vi "Unit Test FGV slit.vi"() -> ()   [LabVIEW 2013]
doc: "Use this template to build a producer/consumer design pattern with events to produce queue items. Use this design pattern instead of the User Interface Event Handler pattern for user interfaces when you want to execute code asynchronously in response to an event without slowing the user interface responsiveness."
uses:
  FGV Slit Data.ctl
  <userlib>/GCSLabView/Low Level/General command.llb/Controller names.ctl
  Action Slit.ctl
  <userlib>/GCSLabView/Low Level/General command.llb/Global2 (Array).vi
panel:
  out "System":T2(array[cluster])
  in  "Initialize":bool
  out "FGV Slit Data Out":T3={"Portnumber"=0, "Position"=0.0, "Status"="", "Système ID"=1, "Connected axes"=[], "Velocity"=0.0, "Stage names"=[], "Device ID out"=0} {"Système ID" min=1 max=10 step=1; "Portnumber" items=["COM1", "COM2", "COM3", "COM4", "COM5", "COM6", "COM7", "COM8", "COM9", "COM10", "COM11", "COM12", "COM13", "COM14", "COM15", "COM16", "COM17", "COM18", "COM19", "COM20", "COM21", "COM22", "COM23", "COM24", "COM25", "COM26", "COM27", "COM28", "COM29", "COM30"]}
  out "Get Velocity":dbl
  in  "Set Velocity":dbl
  in  "Set Velocity":bool
  out "Velocity":dbl
  in  "Get Velocity":bool
  in  "Disconnect":bool
  out "Position Real":dbl
  in  "Move Rel":bool
  in  "Position Rel":dbl
  in  "Position Abs":dbl
  in  "Move Abs":bool
  in  "error in (no error)":errorcluster
  in  "Get Position":bool
  out "error out":errorcluster
  out "Status":string
  in  "Portnumber":i32(ring) items=["COM1", "COM2", "COM3", "COM4", "COM5", "COM6", "COM7", "COM8", "COM9", "COM10", "COM11", "COM12", "COM13", "COM14", "COM15", "COM16", "COM17", "COM18", "COM19", "COM20", "COM21", "COM22", "COM23", "COM24", "COM25", "COM26", "COM27", "COM28", "COM29", "COM30"]
  in  "Connect":bool
  in  "stop":bool
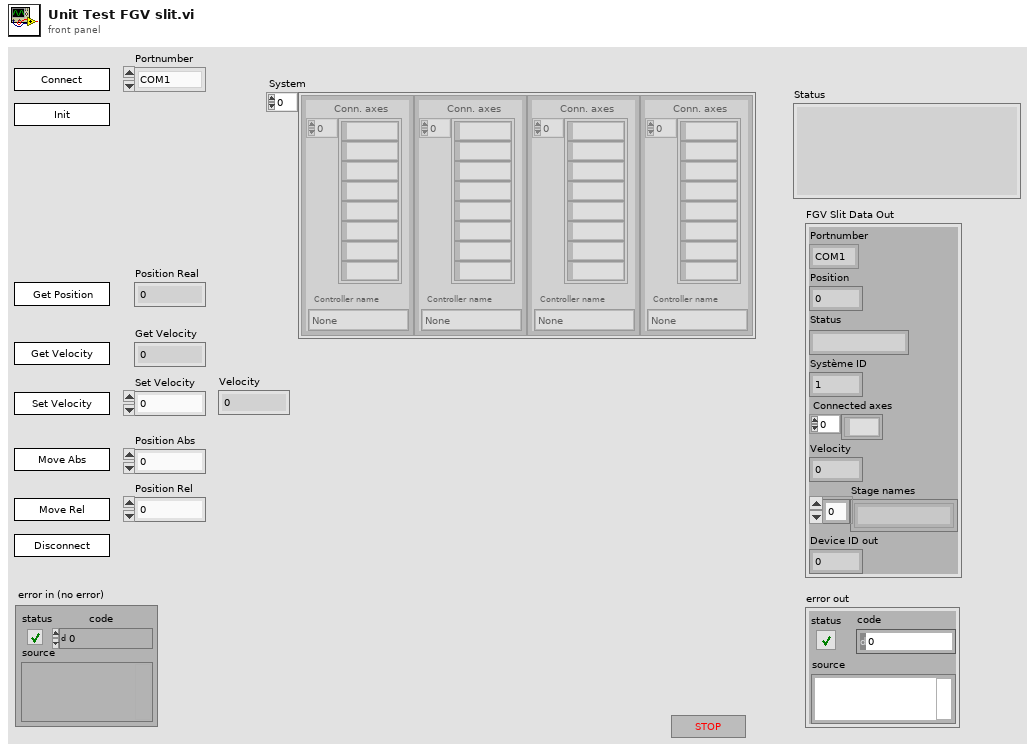
[diagram p1: front panel]
types:
  T1 = typedef "Controller names.ctl" = enum16{"None", "Analog", "C-702", "C-843", "C-843.PM", "C-844", "C-848", "C-865", "C-866", "C-867", "C-880", "E-516", "E-517", "E-709", "E-710", "E-712", "E-725", "E-753", "E-755", "E-761", "E-816", "E-861", "F-206", "M-840", "M-850", "M-8X0", "Mercury", "Mercury_GCS"}
  T2 = cluster{"Conn. axes":string[], "Controller name":T1}[]
  T3 = typedef "FGV Slit Data.ctl" = cluster{"Portnumber":i32, "Position":dbl, "Status":string, "Système ID":i32, "Connected axes":string[], "Velocity":dbl, "Stage names":string[], "Device ID out":i32}
  T4 = typedef "Action Slit.ctl" = enum16{"Connect", "Initialize", "Set Velocity", "Get Velocity", "Move Rel", "Move Abs", "Position", "Status", "Abort", "Disconnect"}
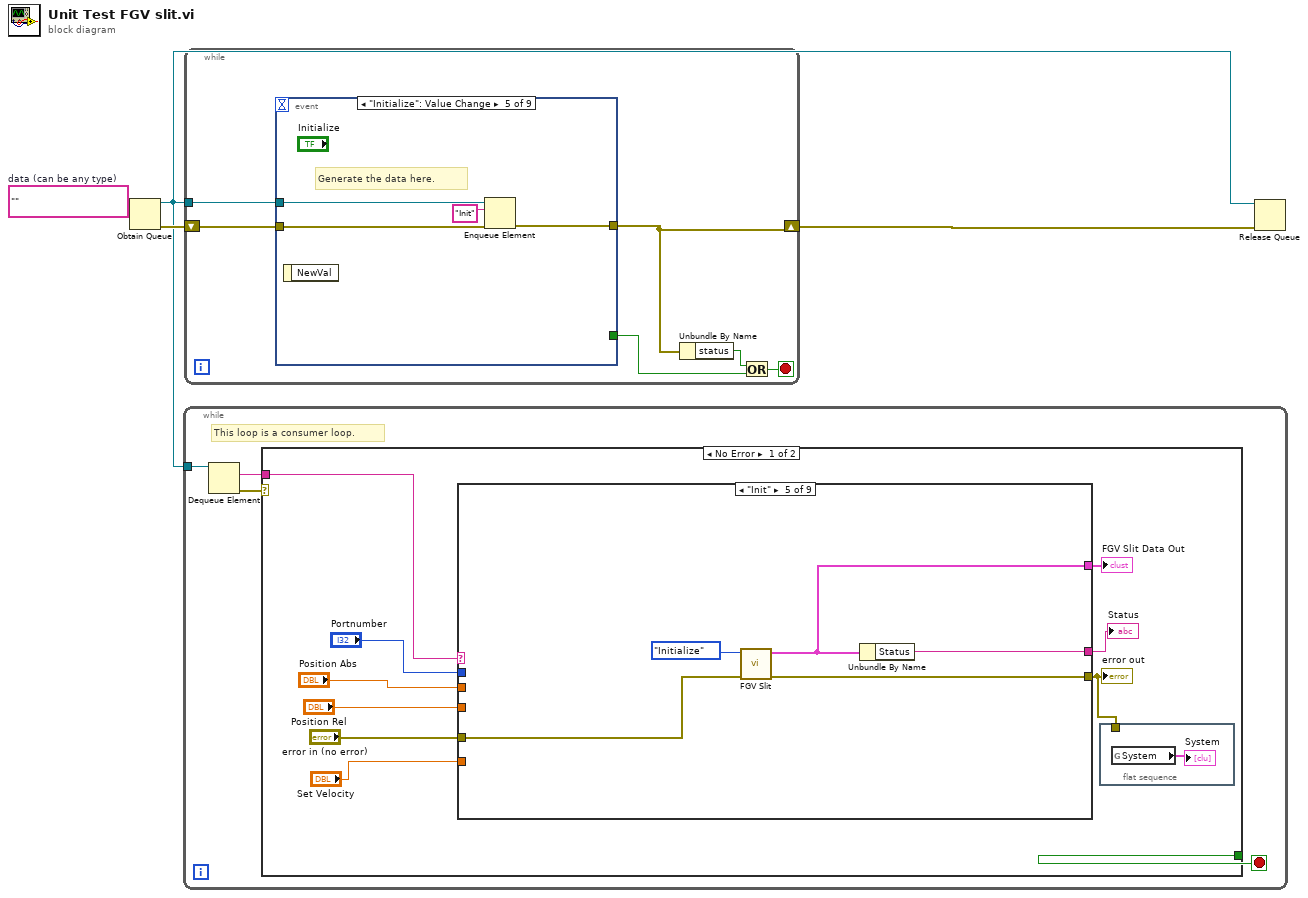
[diagram p0: block diagram]
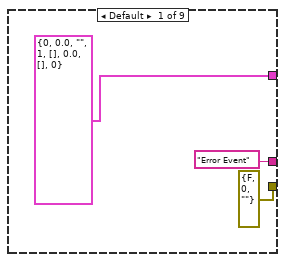
[diagram p2: hidden frame]
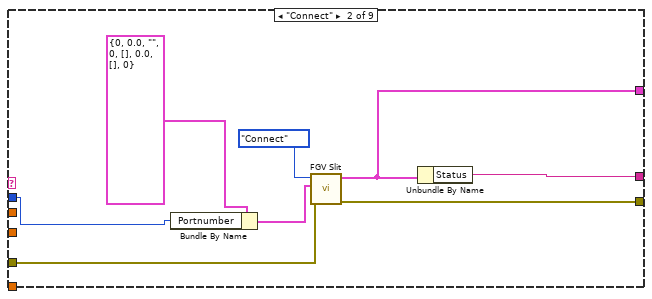
[diagram p3: hidden frame]
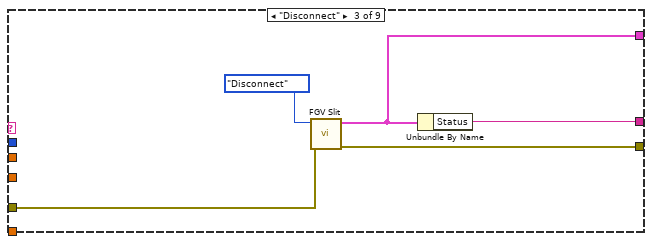
[diagram p4: hidden frame]
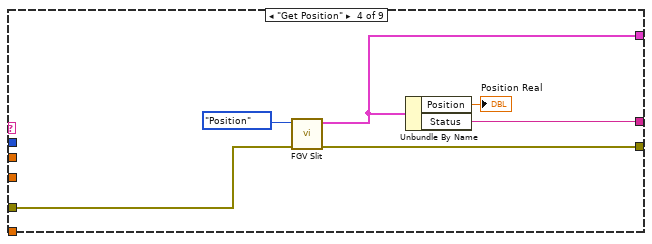
[diagram p5: hidden frame]
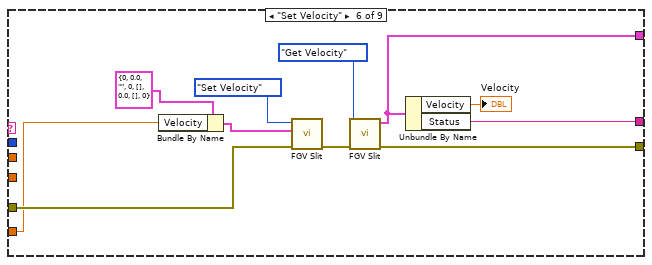
[diagram p6: hidden frame]
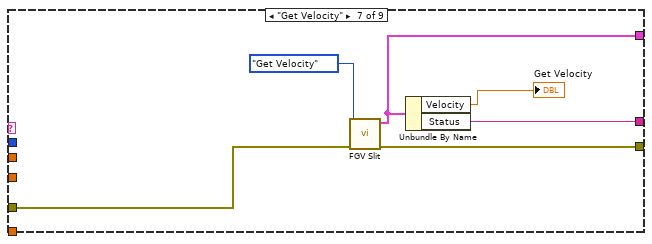
[diagram p7: hidden frame]
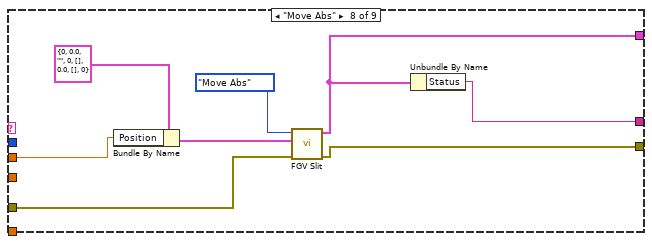
[diagram p8: hidden frame]
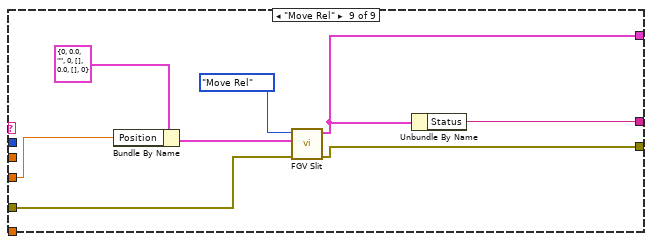
[diagram p9: hidden frame]
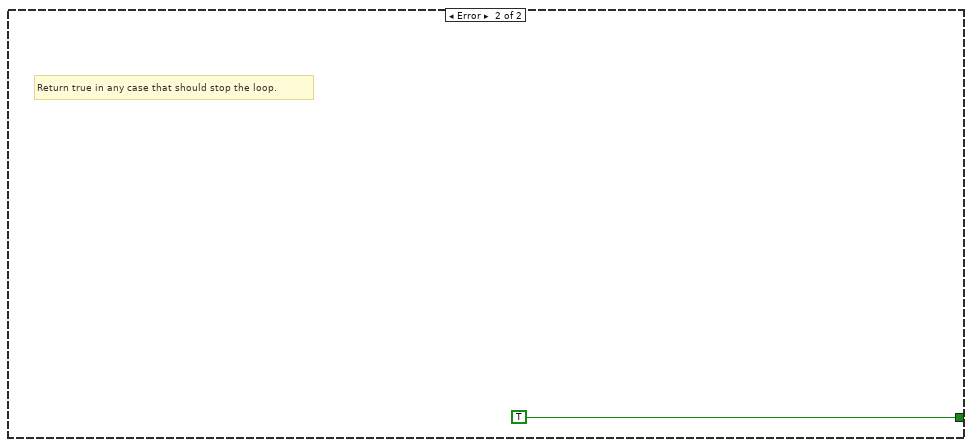
[diagram p10: hidden frame]
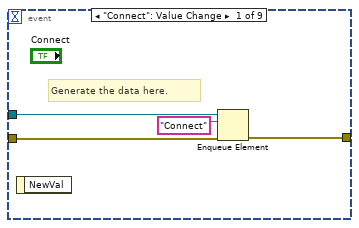
[diagram p11: hidden frame]
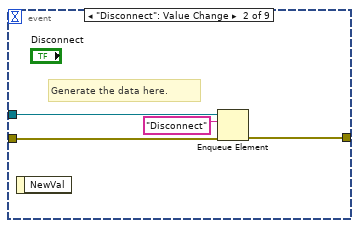
[diagram p12: hidden frame]
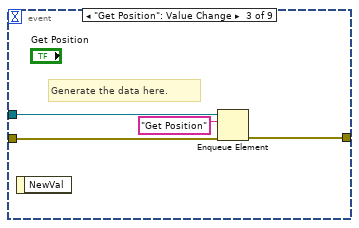
[diagram p13: hidden frame]
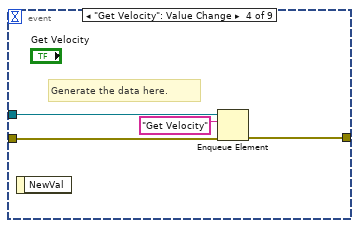
[diagram p14: hidden frame]
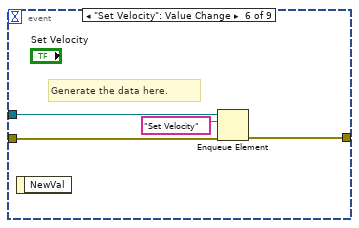
[diagram p15: hidden frame]
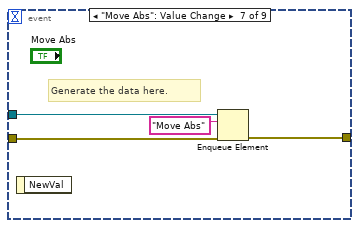
[diagram p16: hidden frame]
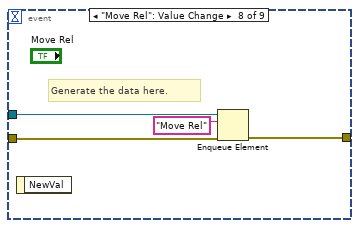
[diagram p17: hidden frame]
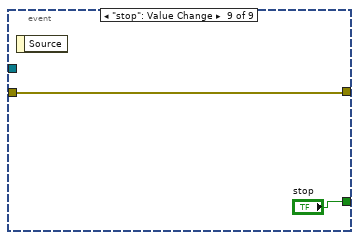
[diagram p18: hidden frame]
diagram:
  w2 = ""  # data (can be any type)
  n1 = Obtain Queue(element data type=w2) -> (queue out=w1:refnum<queue>, error out=w4:errorcluster)  [unwired: 4 in, 1 out]
  n2 = while {
    tunnel: w1 -> [w8]
    stop <- w5 stop-if-true
    # "This loop is a consumer loop."
    n3 = Dequeue Element(queue=w8) -> (element=w6:string, error out=w7:errorcluster)  [unwired: 2 in, 2 out]
    n4 = case shown="No Error" w7 {
      tunnel: w6 -> [w17 _]
      tunnel: [_ TRUE] -> w5
      frame No Error {
        n5 = case shown="\"Init\"" w17 {
          tunnel: "Portnumber" -> [_ w28 _ _ _ _ _ _ _]
          tunnel: ["Error Event" ("Status") w25 w33 w38 w43 w55 w62 w68 w76] -> w15
          tunnel: [errorcluster {"status"=FALSE, "code"=0, "source"=""} ("error out") w24 w32 w39 w44 w48 w61 w69 w77] -> w9
          tunnel: "error in (no error)" -> [_ w23 w31 w37 w42 w54 w59 w67 w75]
          tunnel: "Position Abs" -> [_ _ _ _ _ _ _ w64 _]
          tunnel: "Position Rel" -> [_ _ _ _ _ _ _ _ w72]
          tunnel: "Set Velocity" -> [_ _ _ _ _ w51 _ _ _]
          tunnel: [T3 {"Portnumber"=0, "Position"=0.0, "Status"="", "Système ID"=1, "Connected axes"=[], "Velocity"=0.0, "Stage names"=[], "Device ID out"=0} ("FGV Slit Data Out") w22 w30 w35 w41 w46 w57 w63 w71] -> w10
          frame Default {
          }
          frame "Connect" {
            n6 = Bundle By Name(cluster=T3 {"Portnumber"=0, "Position"=0.0, "Status"="", "Système ID"=0, "Connected axes"=[], "Velocity"=0.0, "Stage names"=[], "Device ID out"=0} ("FGV Slit Data In"), "Portnumber"=w28) -> (w27:T3)
            n7 = call "FGV Slit.vi"("error in (no error)"=w23, "FGV Slit Data In"=w27, "Action"=Action_Slit."Connect") -> ("error out"=w24:errorcluster, "FGV Slit Data Out"=w22:T3)  [unwired: 7 in]
            n8 = Unbundle By Name(w22) -> ("Status"=w25:string)
          }
          frame "Disconnect" {
            n9 = call "FGV Slit.vi"("error in (no error)"=w31, "Action"=Action_Slit."Disconnect") -> ("error out"=w32:errorcluster, "FGV Slit Data Out"=w30:T3)  [unwired: 8 in]
            n10 = Unbundle By Name(w30) -> ("Status"=w33:string)
          }
          frame "Get Position" {
            n11 = call "FGV Slit.vi"("error in (no error)"=w37, "Action"=Action_Slit."Position") -> ("error out"=w39:errorcluster, "FGV Slit Data Out"=w35:T3)  [unwired: 8 in]
            n12 = Unbundle By Name(w35) -> ("Position"=→"Position Real":dbl, "Status"=w38:string)
          }
          frame "Init" {
            n13 = call "FGV Slit.vi"("error in (no error)"=w42, "Action"=Action_Slit."Initialize") -> ("error out"=w44:errorcluster, "FGV Slit Data Out"=w41:T3)  [unwired: 8 in]
            n14 = Unbundle By Name(w41) -> ("Status"=w43:string)
          }
          frame "Set Velocity" {
            n15 = Bundle By Name(cluster=T3 {"Portnumber"=0, "Position"=0.0, "Status"="", "Système ID"=0, "Connected axes"=[], "Velocity"=0.0, "Stage names"=[], "Device ID out"=0} ("FGV Slit Data In"), "Velocity"=w51) -> (w50:T3)
            n16 = call "FGV Slit.vi"("error in (no error)"=w54, "FGV Slit Data In"=w50, "Action"=Action_Slit."Set Velocity") -> ("error out"=w49:errorcluster)  [unwired: 7 in, 1 out]
            n17 = call "FGV Slit.vi"("error in (no error)"=w49, "Action"=Action_Slit."Get Velocity") -> ("error out"=w48:errorcluster, "FGV Slit Data Out"=w46:T3)  [unwired: 8 in]
            n18 = Unbundle By Name(w46) -> ("Velocity"=→"Velocity":dbl, "Status"=w55:string)
          }
          frame "Get Velocity" {
            n19 = call "FGV Slit.vi"("error in (no error)"=w59, "Action"=Action_Slit."Get Velocity") -> ("error out"=w61:errorcluster, "FGV Slit Data Out"=w57:T3)  [unwired: 8 in]
            n20 = Unbundle By Name(w57) -> ("Velocity"=→"Get Velocity":dbl, "Status"=w62:string)
          }
          frame "Move Abs" {
            n21 = Bundle By Name(cluster=T3 {"Portnumber"=0, "Position"=0.0, "Status"="", "Système ID"=0, "Connected axes"=[], "Velocity"=0.0, "Stage names"=[], "Device ID out"=0} ("FGV Slit Data In"), "Position"=w64) -> (w65:T3)
            n22 = call "FGV Slit.vi"("error in (no error)"=w67, "FGV Slit Data In"=w65, "Action"=Action_Slit."Move Abs") -> ("error out"=w69:errorcluster, "FGV Slit Data Out"=w63:T3)  [unwired: 7 in]
            n23 = Unbundle By Name(w63) -> ("Status"=w68:string)
          }
          frame "Move Rel" {
            n24 = Bundle By Name(cluster=T3 {"Portnumber"=0, "Position"=0.0, "Status"="", "Système ID"=0, "Connected axes"=[], "Velocity"=0.0, "Stage names"=[], "Device ID out"=0} ("FGV Slit Data In"), "Position"=w72) -> (w73:T3)
            n25 = call "FGV Slit.vi"("error in (no error)"=w75, "FGV Slit Data In"=w73, "Action"=Action_Slit."Move Rel") -> ("error out"=w77:errorcluster, "FGV Slit Data Out"=w71:T3)  [unwired: 7 in]
            n26 = Unbundle By Name(w71) -> ("Status"=w76:string)
          }
        }
        "Status" <- w15
        "error out" <- w9
        "FGV Slit Data Out" <- w10
        n27 = flat-sequence {
          tunnel: w9 -> [_]
          frame #0 {
            n28 = global read "Global2 (Array).vi" "System"() -> (→"System":T2)
          }
        }
      }
      frame Error {
        # "Return true in any case that should stop the loop."
      }
    }
  }
  n29 = while {
    shift-right: [w81] -> w3
    shift-left: w4 -> [w84]
    tunnel: w1 -> [w85]
    stop <- w82 stop-if-true
    n30 = event shown="[4] \"Initialize\": Value Change" {
      selector: _ -> [_ _ _ _ _ _ _ _ _]
      dyn-events: _ -> [_ _ _ _ _ _ _ _ _]
      timeout: _ -> [_ _ _ _ _ _ _ _ _]
      tunnel: w85 -> [w89 w93 w97 w101 w105 w109 w113 w117 _]
      tunnel: w84 -> [w88 w92 w96 w100 w104 w108 w112 w116 w118]
      tunnel: [w87 w91 w95 w99 w103 w107 w111 w115 w118] -> w81
      tunnel: [_ _ _ _ _ _ _ _ "stop"] -> w83
      event "Connect": Value Change {
        # "Generate the data here."
        n31 = event-data() -> ()  [unwired: 1 in, 1 out]
        n32 = Enqueue Element(queue=w89, element="Connect", error in (no error)=w88) -> (error out=w87:errorcluster)  [unwired: 1 in, 2 out]
      }
      event "Disconnect": Value Change {
        # "Generate the data here."
        n33 = event-data() -> ()  [unwired: 1 in, 1 out]
        n34 = Enqueue Element(queue=w93, element="Disconnect", error in (no error)=w92) -> (error out=w91:errorcluster)  [unwired: 1 in, 2 out]
      }
      event "Get Position": Value Change {
        # "Generate the data here."
        n35 = event-data() -> ()  [unwired: 1 in, 1 out]
        n36 = Enqueue Element(queue=w97, element="Get Position", error in (no error)=w96) -> (error out=w95:errorcluster)  [unwired: 1 in, 2 out]
      }
      event "Get Velocity": Value Change {
        # "Generate the data here."
        n37 = event-data() -> ()  [unwired: 1 in, 1 out]
        n38 = Enqueue Element(queue=w101, element="Get Velocity", error in (no error)=w100) -> (error out=w99:errorcluster)  [unwired: 1 in, 2 out]
      }
      event "Initialize": Value Change {
        # "Generate the data here."
        n39 = event-data() -> ()  [unwired: 1 in, 1 out]
        n40 = Enqueue Element(queue=w105, element="Init", error in (no error)=w104) -> (error out=w103:errorcluster)  [unwired: 1 in, 2 out]
      }
      event "Set Velocity": Value Change {
        # "Generate the data here."
        n41 = event-data() -> ()  [unwired: 1 in, 1 out]
        n42 = Enqueue Element(queue=w109, element="Set Velocity", error in (no error)=w108) -> (error out=w107:errorcluster)  [unwired: 1 in, 2 out]
      }
      event "Move Abs": Value Change {
        # "Generate the data here."
        n43 = event-data() -> ()  [unwired: 1 in, 1 out]
        n44 = Enqueue Element(queue=w113, element="Move Abs", error in (no error)=w112) -> (error out=w111:errorcluster)  [unwired: 1 in, 2 out]
      }
      event "Move Rel": Value Change {
        # "Generate the data here."
        n45 = event-data() -> ()  [unwired: 1 in, 1 out]
        n46 = Enqueue Element(queue=w117, element="Move Rel", error in (no error)=w116) -> (error out=w115:errorcluster)  [unwired: 1 in, 2 out]
      }
      event "stop": Value Change {
        n47 = event-data() -> ()  [unwired: 1 in, 1 out]
      }
    }
    n48 = Unbundle By Name(w81) -> ("status"=w80:bool)
    n49 = Or(x=w80, y=w83) -> (x .or. y?=w82:bool)
  }
  n50 = Release Queue(queue=w1, error in (no error)=w3) -> ()  [unwired: 1 in, 3 out]
